vi "setModbusRxBuffer.vi"(10 "ModbusRxBuffer":refnum<class "ModbusBuffer.lvclass">, 11 "Model in":refnum<class "Model.lvclass">) -> (3 "Model out":refnum<class "Model.lvclass">)   [LabVIEW 2016, in "Model.lvclass"]
uses:
  Model.lvclass
  Common_RT_Modbus/ModbusBuffer/ModbusBuffer.lvclass
  Model.lvclass/Model.ctl
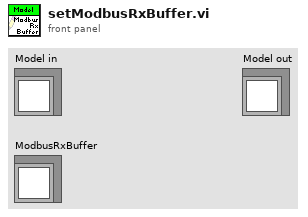
[diagram p1: front panel]
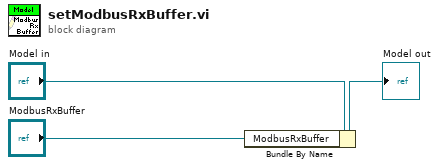
[diagram p0: block diagram]
diagram:
  n1 = Bundle By Name(cluster="Model in", "ModbusRxBuffer"="ModbusRxBuffer") -> (→"Model out":refnum<class "Model.lvclass">)
